vi "Plot Helper (Matrix).vi"(8 "error in (no error)":errorcluster, 9 "offset matrix":sgl[][](array[numeric]), 10 "x matrix":sgl[][](array[numeric])) -> (0 "error out":errorcluster, 3 "3D Plot lvclass Array out":refnum<class "3D Plot Datatype.lvclass">[](array[class]))   [LabVIEW 2020, in "3D Pie Datatype.lvclass"]
doc: "Generates a pie chart."
uses:
  <vilib>/Math Plots/3D Math Plots/3D Pie/3D Pie Datatype/3D Pie Datatype.lvclass
  <vilib>/Math Plots/3D Math Plots/3D Plot/3D Plot Datatype/3D Plot Datatype.lvclass
  e:/builds/penguin/labview/branches/2020/dev/dist/vi.lib/Math Plots/3D Math Plots/3D Plot/3D Plot Datatype/3D Plot Datatype.lvclass
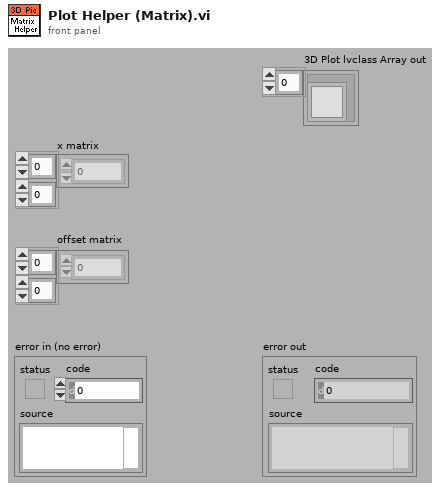
[diagram p1: front panel]
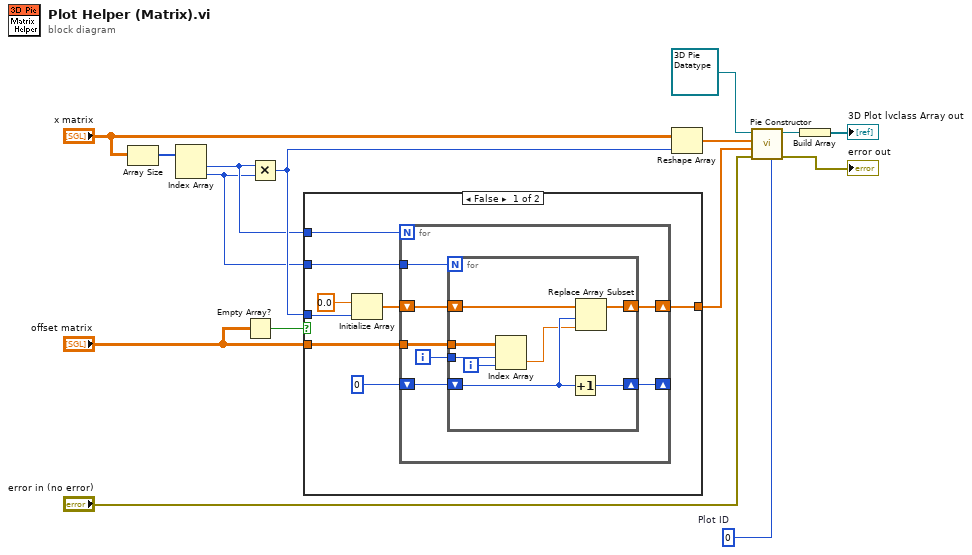
[diagram p0: block diagram]
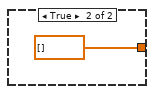
[diagram p2: hidden frame]
diagram:
  w12 = 0  # Plot ID
  n1 = Array Size(array="x matrix") -> (size(s)=w9:i32[])
  n2 = Index Array(array=w9) -> (element #1=w2:i32, element #2=w1:i32)  [unwired: 2 in]
  n3 = Empty Array?(array="offset matrix") -> (empty?=w6:bool)
  n4 = Multiply(x=w2, y=w1) -> (x*y=w4:i32)
  n5 = case shown="False" w6 {
    tunnel: [w20 sgl[] [] ("output array")] -> w5
    tunnel: w4 -> [w22 _]
    tunnel: "offset matrix" -> [w18 _]
    tunnel: w2 -> [w17 _]
    tunnel: w1 -> [w16 _]
    frame False {
      n6 = Initialize Array(sgl 0.0, w22) -> (w21:sgl[])
      n7 = for {
        N: w17 -> [_]
        shift-right: [w29] -> w20
        shift-left: w21 -> [w30]
        shift-right: [w27] -> _
        shift-left: 0 -> [w28]
        tunnel: w18 -> [w26]
        tunnel: w16 -> [w24]
        i -> [w25]
        n8 = for {
          N: w24 -> [_]
          shift-right: [w37] -> w29
          shift-left: w30 -> [w38]
          shift-right: [w35] -> w27
          shift-left: w28 -> [w36]
          tunnel: w26 -> [w34]
          tunnel: w25 -> [w33]
          i -> [w32]
          n9 = Index Array(array=w34, index (row)=w33, index (col)=w32) -> (element=w31:sgl)
          n10 = Increment(x=w36) -> (x+1=w35:i32)
          n11 = Replace Array Subset(array=w38, new element=w31, index=w36) -> (w37:sgl[])
        }
      }
    }
    frame True {
    }
  }
  n12 = Reshape Array("x matrix", w4) -> (w8:sgl[])
  n13 = call <vilib>:"Pie Constructor.vi"("Plot ID"=w12, "error in (no error)"="error in (no error)", "offset vector"=w5, "x vector"=w8, "3D Quiver Datatype.lvclass in"=refnum<class "3D Pie Datatype.lvclass"> refnum) -> ("error out"=→"error out":errorcluster, "3D Quiver Datatype.lvclass out"=w11:refnum<class "3D Pie Datatype.lvclass">)  [unwired: 5 out]
  n14 = Build Array(w11) -> (→"3D Plot lvclass Array out":refnum<class "3D Pie Datatype.lvclass">[])
